vi "NI PostMessage Master.vi"(8 "error in (no error)":errorcluster, 10 "function":T1(ring)=enum."Start Screen Saver", 11 "window refnum":refnum<k1>) -> (0 "error out":errorcluster)   [LabVIEW 2018]
doc: "This VI acts as a \"Master\" for various VIs that use the LVPostMessage function in the LVWUTIL.DLL library. This is basically just the PostMessage API function with a WM_SYSCOMMAND message, but also does some additional checking for the existance of the targeted window."
uses:
  LVWUtil32.dll
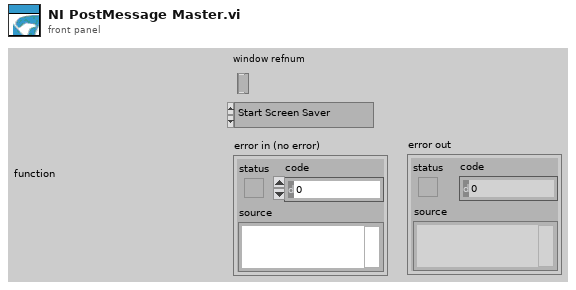
[diagram p1: front panel]
types:
  T1 = enum8{"Maximize Window", "Minimize Window", "Show Task List", "Start Screen Saver", "Quit Application"}
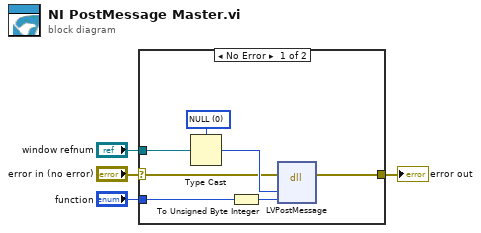
[diagram p0: block diagram]
diagram:
  n1 = case shown="No Error" "error in (no error)" {
    selector: "error in (no error)" -> [w7 w12]
    tunnel: "window refnum" -> [w8 _]
    tunnel: "function" -> [w6 _]
    tunnel: [w5 w12] -> w1
    frame No Error {
      w9 = u32 0 items=["NULL"]
      n2 = Type Cast(type=w9, x=w8) -> (*(type *) &x=w10:u32)
      n3 = To Unsigned Byte Integer(number=w6) -> (unsigned 8bit integer=w11:u8)
      n4 = dll-call lib="C:/Users/John Gmitter/OneDrive - National Instruments/Projects/Harris FL/Manticore/Harris SW upgrades/Reference Management Server/Generic Reuse/Windows Utilities/LVWUtil32.DLL" fn="LVPostMessage"(error in=w7, "hWnd"=w10, "function"=w11) -> (error out=w5:errorcluster)  [unwired: 5 in, 1 out]
    }
    frame Error {
    }
  }
  "error out" <- w1
